vi "JKI Prompt Web Browser Path__jki_lib_communication -- VI Tester.vi"(4 "error in (no error)":errorcluster) -> (0 "error out":errorcluster, 3 "browser path":string)   [LabVIEW 2011]
panel:
  in  "prompt":string="Please select your Web Browser"
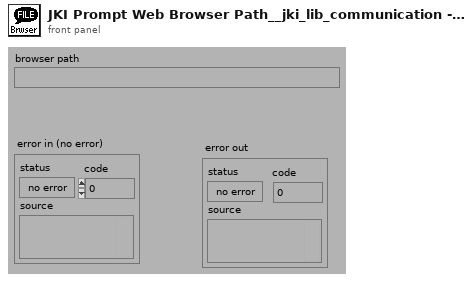
[diagram p1: front panel]
types:
  T1 = enum16{"read/write", "read-only", "write-only", "write-only (truncate)"}
  T2 = enum16{"existing file", "new file", "new or existing file", "existing dir", "new dir", "new or existing dir"}
  T3 = enum16{"open", "replace", "create", "open or create", "replace or create", "replace or create with confirmation"}
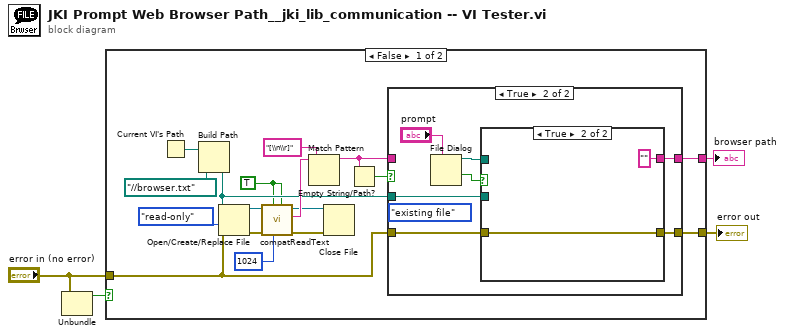
[diagram p0: block diagram]
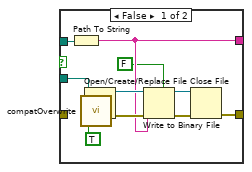
[diagram p3: hidden frame]
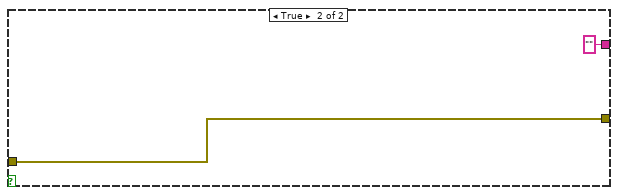
[diagram p4: hidden frame]
diagram:
  n1 = Unbundle("error in (no error)") -> ("status"=w1:bool)  [unwired: 2 out]
  n2 = case shown="False" w1 {
    tunnel: "error in (no error)" -> [w21 w45]
    tunnel: [w17 "" ("before substring")] -> w3
    tunnel: [w15 w45] -> w4
    frame False {
      w11 = TRUE ("line mode (F)")
      n3 = Current VI's Path() -> (path=w5:path)
      n4 = Build Path(base path=w5, name or relative path=path "../../browser.txt") -> (appended path=w16:path)
      n5 = Open/Create/Replace File(file path (use dialog)=w16, error in=w21, access (0:read/write)=T1."read-only" ("open mode (0)")) -> (refnum out=w8:refnum<file>, error out=w9:errorcluster)  [unwired: 3 in, 1 out]
      n6 = call <vilib>:"compatReadText.vi"("convert eol (F)"=w11, "count"=1024, "line mode (F)"=w11, "error in"=w9, "refnum"=w8) -> ("error out"=w12:errorcluster, "data"=w20:string, "dup refnum"=w13:refnum<file>)  [unwired: 4 in]
      n7 = Match Pattern(string=w20, regular expression="[\\n\\r]") -> (before substring=w19:string)  [unwired: 1 in, 3 out]
      n8 = Close File(refnum=w13, error in=w12) -> ()  [unwired: 2 out]
      n9 = Empty String/Path?(string/path=w19) -> (empty?=w14:bool)
      n10 = case shown="True" w14 {
        tunnel: w21 -> [w22 w29]
        tunnel: [w22 w28] -> w15
        tunnel: w16 -> [_ w27]
        tunnel: [w23 w25] -> w17
        tunnel: w19 -> [w23 _]
        frame False {
        }
        frame True {
          (unwired) T2."existing file" ("select mode (2)")
          n11 = File Dialog(7:"prompt") -> (1:w30:bool, 3:w26:path)  [unwired: 6 in, 2 out]
          n12 = case shown="True" w30 {
            tunnel: w29 -> [_ w43]
            tunnel: [w34 w43] -> w28
            tunnel: w27 -> [w41 _]
            tunnel: w26 -> [w37 _]
            tunnel: [w33 ""] -> w25
            frame False {
              n13 = Path To String(path=w37) -> (string=w33:string)
              n14 = call <vilib>:"compatOverwrite.vi"("overwrite (F)"=TRUE) -> ("overwrite?"=w31:T3)
              n15 = Open/Create/Replace File(file path (use dialog)=w41, operation (0:open)=w31) -> (refnum out=w38:refnum<file>, error out=w39:errorcluster)  [unwired: 4 in, 1 out]
              n16 = Write to Binary File(file (use dialog)=w38, data=w33, error in=w39, 5:FALSE ("prepend array or string size? (T)")) -> (refnum out=w35:refnum<file>, error out=w36:errorcluster)  [unwired: 2 in, 1 out]
              n17 = Close File(refnum=w35, error in=w36) -> (error out=w34:errorcluster)  [unwired: 1 out]
            }
            frame True {
            }
          }
        }
      }
    }
    frame True {
    }
  }
  "error out" <- w4
  "browser path" <- w3
